vi "Actor Core.vi"(8 "error in":errorcluster, 11 "CS++GoBangClient in":refnum<class "CS++GoBangClient.lvclass">) -> (0 "error out":errorcluster, 3 "Actor out":refnum<class "Actor.lvclass">)   [LabVIEW 2013, in "GoBang.lvlib" / "CS++GoBangClient.lvclass"]
doc: "(<B>Filename</B>: Actor Framework.lvlib:Actor.lvclass:Actor Core.vi)\n\nReceives messages to the actor, reacts to them, and initiates any error handling that may shut the actor down.\n\nDescendant classes may override this VI to append parallel tasks for the actor to complete while it handles messages. Overrides use the Call Parent Method node."
uses:
  CS++GoBangClient.lvclass
  <vilib>/ActorFramework/Actor/Actor.lvclass
  typdefs/BoardField.ctl
  typdefs/GameState.ctl
  Core/Actors/CS++SVMonitor/CS++SVMonitor.lvclass
  CS++GoBangClient Messages/Write black player Msg/Write black player Msg.lvclass
  CS++GoBangClient Messages/Write white player Msg/Write white player Msg.lvclass
  CS++GoBangClient Messages/Write game board Msg/Write game board Msg.lvclass
  CS++GoBangClient Messages/Write game state Msg/Write game state Msg.lvclass
  Core/Actors/CS++BaseActor/CS++BaseActor.lvclass/CS++BaseActor.ctl
  <vilib>/ActorFramework/Actor/Actor.lvclass/Actor.ctl
  <vilib>/ActorFramework/Message Enqueuer/Message Enqueuer.lvclass/Message Enqueuer.ctl
  CS++GoBangClient.lvclass/CS++GoBangClient.ctl
  Core/Actors/CS++PVMonitor/CS++PVMonitor.lvclass/CS++PVMonitor.ctl
  Core/Actors/CS++PVMonitor Messages/Register PVs Msg/Register PVs Msg.lvclass/Register PVs Msg.ctl
  CS++GoBangClient Messages/Send Move Msg/Send Move Msg.lvclass/Send Move Msg.ctl
  CS++GoBangClient Messages/Join Game Msg/Join Game Msg.lvclass/Join Game Msg.ctl
  Core/Actors/CS++BaseActor/CS++BaseActor.lvclass
  <vilib>/ActorFramework/Message Enqueuer/Init from Existing Queue.vi
  <vilib>/ActorFramework/Message Enqueuer/Enqueue.vi
  <vilib>/ActorFramework/Message Priority Queue/Priority Enqueue.vi
  <vilib>/ActorFramework/Message Enqueuer/Message Enqueuer.lvclass
  Core/Actors/CS++PVMonitor Messages/Register PVs Msg/Register PVs Msg.lvclass
  CS++GoBangClient Messages/Send Move Msg/Send Move Msg.lvclass
  CS++GoBangClient Messages/Join Game Msg/Join Game Msg.lvclass
  <vilib>/ActorFramework/Stop Msg/Stop Msg.lvclass
  GoBang.lvlib
  Core/Actors/CS++PVMonitor/CS++PVMonitor.lvclass
  Core/Classes/CS++ProcessVariables/PVConnection/PVConnection.lvclass
panel:
  in  "OppColor":T1
  out "Opponnents name":string
  in  "Color":T1
  in  "Your name":string
  in  "stone":T1
  in  "stop":bool
  in  "State":T2
  out "GameBoard":T1[][](array[typedef])
  out "White won":bool
  out "Black won":bool
  out "Game over":bool
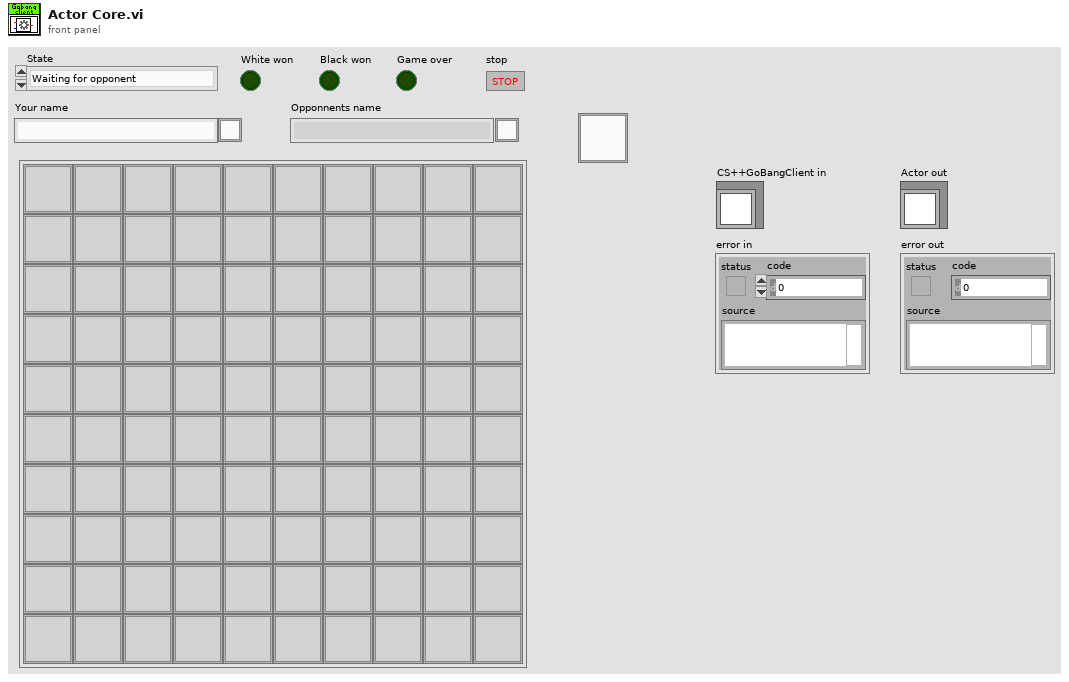
[diagram p1: front panel]
types:
  T1 = typedef "GoBang.lvlib/BoardField.ctl" = u8
  T2 = typedef "GoBang.lvlib/GameState.ctl" = enum16{"Waiting for opponent", "White to move", "Black to move", "Game over, white won", "Game over, black won"}
  T3 = enum32{"Invalid", "Standard", "Closed", "Hidden", "Minimized", "Maximized"}
  T4 = cluster{"BlackPlayer":string, "GoBang.lvlib:Write black player Msg.lvclass":refnum<class "Write black player Msg.lvclass">}
  T5 = cluster{"GameBoard":string, "GoBang.lvlib:Write game board Msg.lvclass":refnum<class "Write game board Msg.lvclass">}
  T6 = cluster{"GameState":string, "GoBang.lvlib:Write game state Msg.lvclass":refnum<class "Write game state Msg.lvclass">}
  T7 = cluster{"WhitePlayer":string, "GoBang.lvlib:Write white player Msg.lvclass":refnum<class "Write white player Msg.lvclass">}
  T8 = cluster{"GameState":string, "GoBang.lvlib:Write white player Msg.lvclass":refnum<class "CS++PVUpdate Msg.lvclass">}[]
  T9 = cluster{"Self Enqueuer":refnum<class "Message Enqueuer.lvclass">, cluster{"GameState":string, "GoBang.lvlib:Write white player Msg.lvclass":refnum<class "CS++PVUpdate Msg.lvclass">}[]}
  T10 = typedef "LVPositionTypeDef.ctl" = cluster{"Left":i32, "Top":i32}
  T11 = typedef "LVBoundsTypeDef.ctl" = cluster{"Width":u32, "Height":u32}
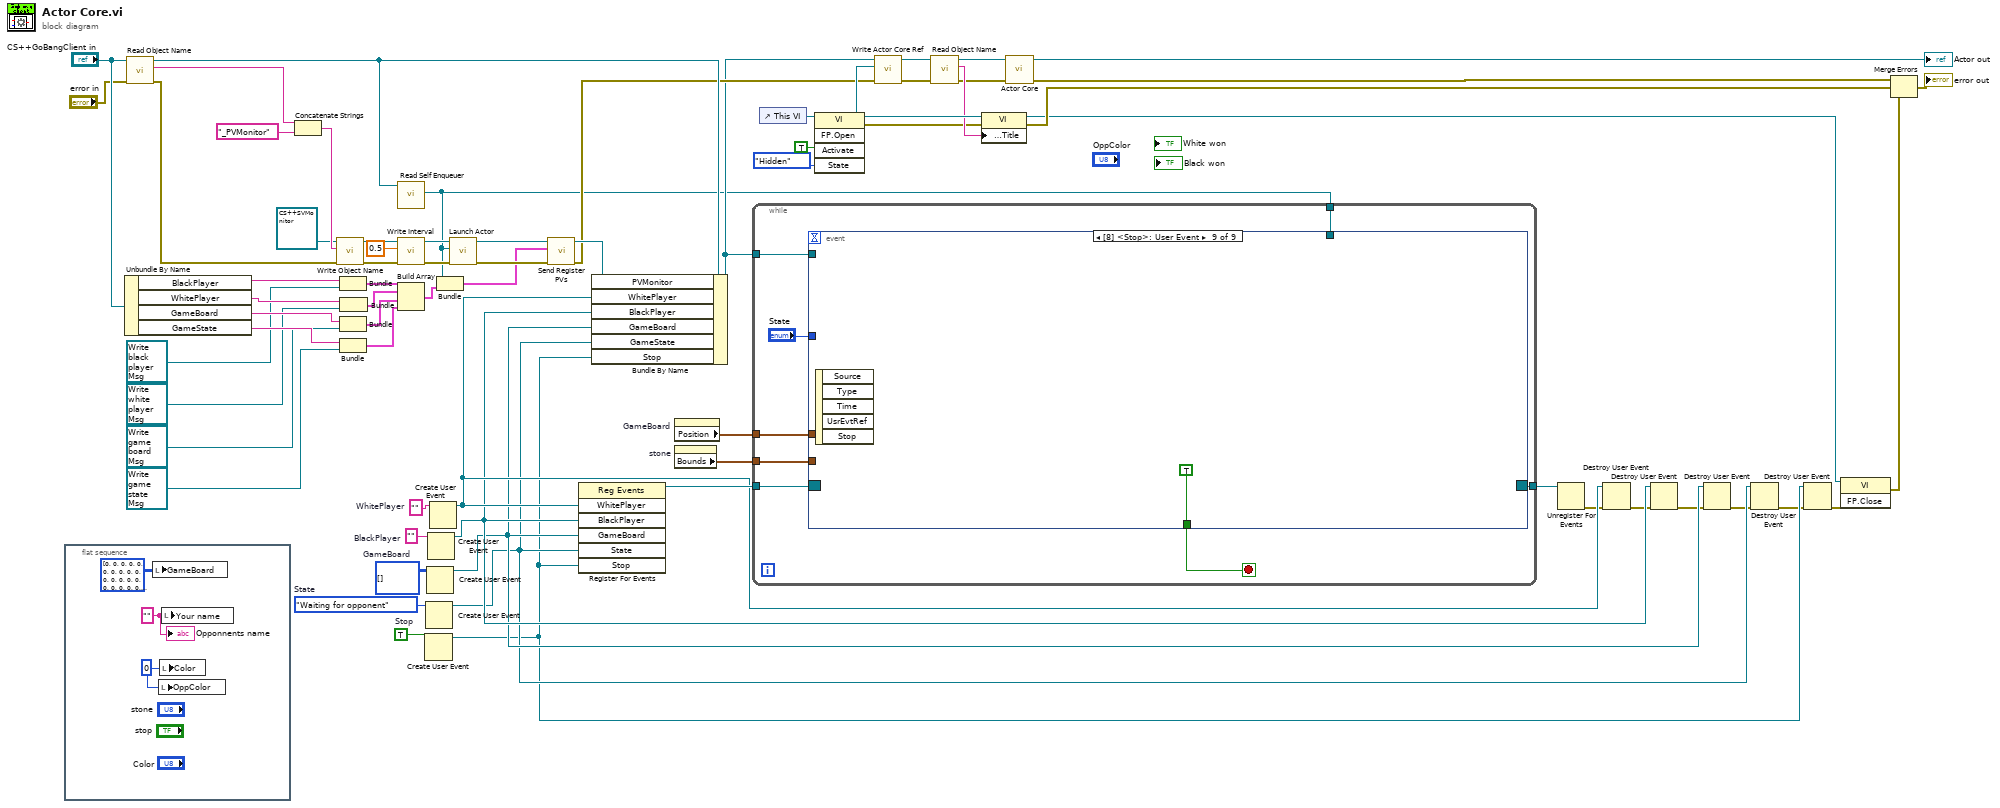
[diagram p0: block diagram]
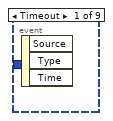
[diagram p2: hidden frame]
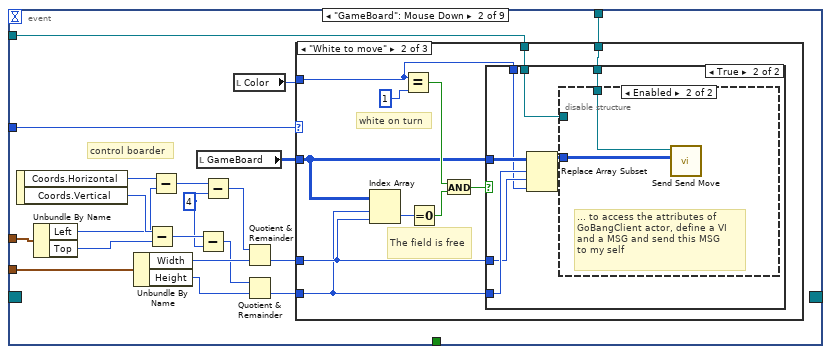
[diagram p3: hidden frame]
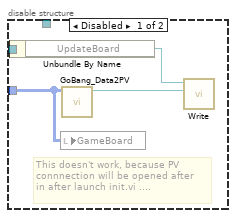
[diagram p6: hidden frame]
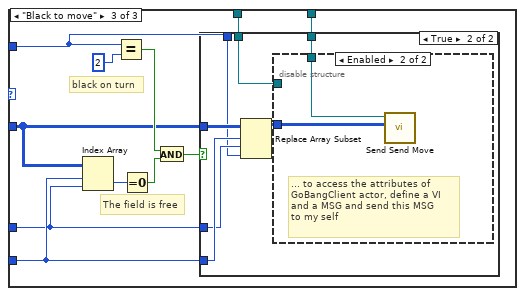
[diagram p7: hidden frame]
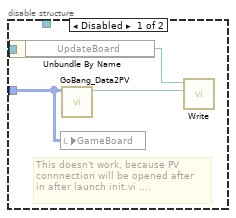
[diagram p9: hidden frame]
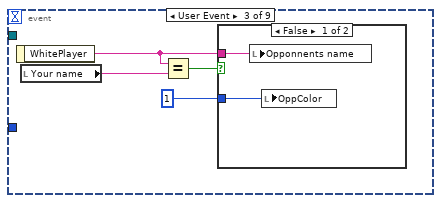
[diagram p10: hidden frame]
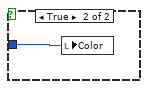
[diagram p11: hidden frame]
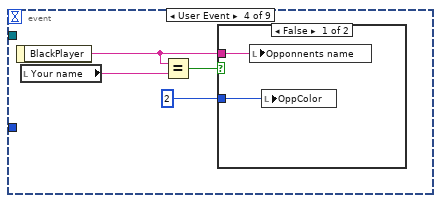
[diagram p12: hidden frame]
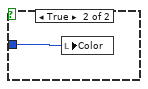
[diagram p13: hidden frame]
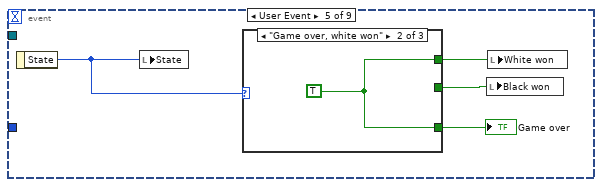
[diagram p14: hidden frame]
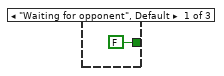
[diagram p15: hidden frame]
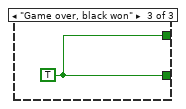
[diagram p16: hidden frame]
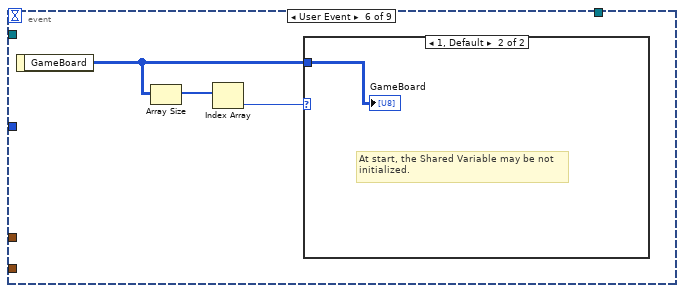
[diagram p17: hidden frame]
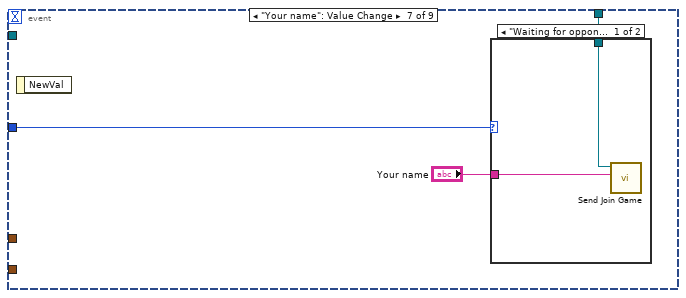
[diagram p19: hidden frame]
diagram:
  w32 = TRUE  # Stop
  w39 = T1[][] []  # GameBoard
  w40 = GameState."Waiting for opponent"  # State
  w41 = ""  # BlackPlayer
  w42 = ""  # WhitePlayer
  n1 = flat-sequence {
    frame #0 {
      w70 = T1 0 ("Color")
      w69 = "" ("Your name")
      n2 = local write "GameBoard"(T1[][] [[0, 0, 0, 0, 0, 0, 0, 0, 0, 0], [0, 0, 0, 0, 0, 0, 0, 0, 0, 0], [0, 0, 0, 0, 0, 0, 0, 0, 0, 0], [0, 0, 0, 0, 0, 0, 0, 0, 0, 0], [0, 0, 0, 0, 0, 0, 0, 0, 0, 0], [0, 0, 0, 0, 0, 0, 0, 0, 0, 0], [0, 0, 0, 0, 0, 0, 0, 0, 0, 0], [0, 0, 0, 0, 0, 0, 0, 0, 0, 0], [0, 0, 0, 0, 0, 0, 0, 0, 0, 0], [0, 0, 0, 0, 0, 0, 0, 0, 0, 0]] ("GameBoard")) -> ()
      n3 = local write "OppColor"(w70) -> ()
      n4 = local write "Color"(w70) -> ()
      n5 = local write "Your name"(w69) -> ()
      "Opponnents name" <- w69
    }
  }
  n6 = Unbundle By Name("CS++GoBangClient in") -> ("BlackPlayer"=w64:string, "WhitePlayer"=w48:string, "GameBoard"=w47:string, "GameState"=w46:string)
  n7 = call "Read Object Name.vi"("error in (no error)"="error in", "CS++BaseActor in"="CS++GoBangClient in") -> ("error out"=w19:errorcluster, "Object Name"=w50:string, "CS++BaseActor out"=w33:refnum<class "CS++GoBangClient.lvclass">)  [unwired: 7 in]
  n8 = Concatenate Strings(w50, "_PVMonitor" ("Object Name")) -> (w58:string)
  n9 = call "Write Object Name.vi"("error in (no error)"=w19, "Object Name"=w58, "CS++BaseActor in"=refnum<class "CS++SVMonitor.lvclass"> refnum ("CS++SVMonitor.lvlib:CS++SVMonitor.lvclass")) -> ("error out"=w55:errorcluster, "CS++BaseActor out"=w57:refnum<class "CS++SVMonitor.lvclass">)  [unwired: 7 in]
  n10 = Bundle("BlackPlayer"=w64, "GoBang.lvlib:Write black player Msg.lvclass"=refnum<class "Write black player Msg.lvclass"> refnum) -> (w63:T4)  [unwired: 1 in]
  n11 = Bundle("GameBoard"=w47, "GoBang.lvlib:Write game board Msg.lvclass"=refnum<class "Write game board Msg.lvclass"> refnum) -> (w44:T5)  [unwired: 1 in]
  n12 = Bundle("GameState"=w46, "GoBang.lvlib:Write game state Msg.lvclass"=refnum<class "Write game state Msg.lvclass"> refnum) -> (w43:T6)  [unwired: 1 in]
  n13 = Bundle("WhitePlayer"=w48, "GoBang.lvlib:Write white player Msg.lvclass"=refnum<class "Write white player Msg.lvclass"> refnum) -> (w45:T7)  [unwired: 1 in]
  n14 = call <vilib>:"Read Self Enqueuer.vi"("Actor"=w33) -> ("Self Enqueuer"=w5:refnum<class "Message Enqueuer.lvclass">)  [unwired: 10 in]
  n15 = call "Write Interval.vi"("error in (no error)"=w55, "Interval"=dbl[unit] 0.5, "CS++PVMonitor in"=w57) -> ("error out"=w51:errorcluster, "CS++PVMonitor out"=w59:refnum<class "CS++SVMonitor.lvclass">)  [unwired: 7 in]
  n16 = Build Array(w63, w45, w44, w43) -> (w62:T8)
  n17 = Create User Event(user event datatype=w32) -> (user event=w12:refnum<user-event>)  [unwired: 1 in, 1 out]
  n18 = Create User Event(user event datatype=w40) -> (user event=w13:refnum<user-event>)  [unwired: 1 in, 1 out]
  n19 = Create User Event(user event datatype=w39) -> (user event=w14:refnum<user-event>)  [unwired: 1 in, 1 out]
  n20 = Create User Event(user event datatype=w41) -> (user event=w15:refnum<user-event>)  [unwired: 1 in, 1 out]
  n21 = Create User Event(user event datatype=w42) -> (user event=w16:refnum<user-event>)  [unwired: 1 in, 1 out]
  n22 = Bundle("Self Enqueuer"=w5, w62) -> (w53:T9)  [unwired: 1 in]
  n23 = call <vilib>:"Launch Actor.vi"("error in (no error)"=w51, "Actor-to-Caller Enqueuer"=w5, "Actor"=w59) -> ("error out"=w54:errorcluster, "Caller-To-Actor Enqueuer"=w52:refnum<class "Message Enqueuer.lvclass">)  [unwired: 7 in]
  n24 = call "Send Register PVs.vi"("error in (no error)"=w54, "Register Info"=w53, "Message Enqueuer"=w52) -> ("error out"=w18:errorcluster)  [unwired: 7 in, 1 out]
  n25 = register-events(w16, w15, w14, w13, w12) -> (reference out=w38:refnum<event-registration>)  [unwired: 2 in, 1 out]
  n26 = Bundle By Name(cluster=w33, "PVMonitor"=w52, "WhitePlayer"=w16, "BlackPlayer"=w15, "GameBoard"=w14, "GameState"=w13, "Stop"=w12) -> (w6:refnum<class "CS++GoBangClient.lvclass">)
  n27 = property on="GameBoard" class="Arr (strict)"() -> ("Position"=w65:T10)  [unwired: 2 in, 2 out]
  n28 = property on="stone" class="Ring (strict)"() -> ("Bounds"=w66:T11)  [unwired: 2 in, 2 out]
  n29 = while {
    tunnel: w66 -> [w78]
    tunnel: w65 -> [w77]
    tunnel: w38 -> [w76]
    tunnel: w6 -> [w75]
    tunnel: [w73] -> w17
    tunnel: w5 -> [w72]
    stop <- w79 stop-if-true
    n30 = event shown="[8] <Stop>: User Event" {
      selector: w76 -> [_ _ _ _ _ _ _ _ _]
      dyn-events: [_ _ _ _ _ _ _ _ _] -> w73
      timeout: _ -> [_ _ _ _ _ _ _ _ _]
      tunnel: [_ _ _ _ _ _ _ TRUE TRUE] -> w79
      tunnel: w78 -> [_ w99 _ _ _ _ _ _ _]
      tunnel: w77 -> [_ w94 _ _ _ _ _ _ _]
      tunnel: w75 -> [_ w81 _ _ _ _ _ w180 _]
      tunnel: "State" -> [_ w84 _ _ _ _ w175 _ _]
      tunnel: w72 -> [_ w80 _ _ _ _ w173 _ _]
      event Timeout {
        n31 = event-data() -> ()  [unwired: 1 in, 3 out]
      }
      event "GameBoard": Mouse Down {
        w87 = 4 ("y 2")
        # "control boarder"
        n32 = event-data() -> ("Coords.Horizontal"=w98:i32, "Coords.Vertical"=w96:i32)  [unwired: 1 in]
        n33 = Unbundle By Name(w94) -> ("Left"=w93:i32, "Top"=w92:i32)
        n34 = Unbundle By Name(w99) -> ("Width"=w97:u32, "Height"=w95:u32)
        n35 = Subtract(x=w96, y=w92) -> (x-y=w90:i32)
        n36 = Subtract(x=w98, y=w93) -> (x-y=w91:i32)
        n37 = local read "GameBoard"() -> (w83:T1[][])
        n38 = Subtract(x=w90, y=w87) -> (x-y=w88:i32)
        n39 = Subtract(x=w91, y=w87) -> (x-y=w89:i32)
        n40 = local read "Color"() -> (w82:T1)
        n41 = Quotient & Remainder(x=w89, y=w97) -> (floor(x/y)=w86:u32)  [unwired: 1 out]
        n42 = Quotient & Remainder(x=w88, y=w95) -> (floor(x/y)=w85:u32)  [unwired: 1 out]
        n43 = case shown="\"White to move\"" w84 {
          tunnel: w86 -> [_ w102 w133]
          tunnel: w85 -> [_ w101 w134]
          tunnel: w83 -> [_ w104 w128]
          tunnel: w82 -> [_ w100 w126]
          tunnel: w81 -> [_ w105 w125]
          tunnel: w80 -> [_ w106 w124]
          frame "Waiting for opponent", Default {
          }
          frame "White to move" {
            # "white on turn"
            # "The field is free"
            n44 = Index Array(array=w104, index (row)=w101, index (col)=w102) -> (element=w110:T1)
            n45 = Equal?(x=w100, y=T1 1) -> (x = y?=w108:bool)
            n46 = Equal To 0?(x=w110) -> (x = 0?=w109:bool)
            n47 = And(x=w108, y=w109) -> (x .and. y?=w103:bool)
            n48 = case shown="True" w103 {
              tunnel: w101 -> [_ w117]
              tunnel: w102 -> [_ w116]
              tunnel: w104 -> [_ w115]
              tunnel: w100 -> [_ w114]
              tunnel: w105 -> [_ w112]
              tunnel: w106 -> [_ w111]
              frame False {
              }
              frame True {
                n49 = Replace Array Subset(array=w115, new element=w114, index (row)=w117, index (col)=w116) -> (w113:T1[][])
                n50 = disable-structure shown="Enabled" {
                  disable-tunnel: w113 -> [w120 w122]
                  disable-tunnel: w112 -> [w118 _]
                  disable-tunnel: w111 -> [_ w123]
                  frame Disabled {
                    # "This doesn't work, because PV\nconnnection will be opened after\nin after launch init.vi ...."
                    n51 = Unbundle By Name(w118) -> ("UpdateBoard"=w119:refnum<class "PVConnection.lvclass">)
                    n52 = local write "GameBoard"(w120) -> ()
                    n53 = call "GoBang_Data2PV.vi"("Data in"=w120) -> ("PV out"=w121:refnum<class "PV.lvclass">)  [unwired: 10 in]
                    n54 = call-dynamic "Write.vi"("PV"=w121, "PVConnection in"=w119) -> ()  [unwired: 8 in, 2 out]
                  }
                  frame Enabled {
                    # "... to access the attributes of \nGoBangClient actor, define a VI \nand a MSG and send this MSG \nto my self"
                    n55 = call "Send Send Move.vi"("GameBoard"=w122, "Message Enqueuer"=w123) -> ()  [unwired: 8 in, 2 out]
                  }
                }
              }
            }
          }
          frame "Black to move" {
            # "black on turn"
            # "The field is free"
            n56 = Index Array(array=w128, index (row)=w134, index (col)=w133) -> (element=w132:T1)
            n57 = Equal?(x=w126, y=T1 2) -> (x = y?=w129:bool)
            n58 = Equal To 0?(x=w132) -> (x = 0?=w130:bool)
            n59 = And(x=w129, y=w130) -> (x .and. y?=w131:bool)
            n60 = case shown="True" w131 {
              tunnel: w134 -> [_ w141]
              tunnel: w133 -> [_ w140]
              tunnel: w128 -> [_ w139]
              tunnel: w126 -> [_ w138]
              tunnel: w125 -> [_ w136]
              tunnel: w124 -> [_ w135]
              frame False {
              }
              frame True {
                n61 = Replace Array Subset(array=w139, new element=w138, index (row)=w141, index (col)=w140) -> (w137:T1[][])
                n62 = disable-structure shown="Enabled" {
                  disable-tunnel: w137 -> [w144 w146]
                  disable-tunnel: w136 -> [w142 _]
                  disable-tunnel: w135 -> [_ w147]
                  frame Disabled {
                    # "This doesn't work, because PV\nconnnection will be opened after\nin after launch init.vi ...."
                    n63 = Unbundle By Name(w142) -> ("UpdateBoard"=w143:refnum<class "PVConnection.lvclass">)
                    n64 = local write "GameBoard"(w144) -> ()
                    n65 = call "GoBang_Data2PV.vi"("Data in"=w144) -> ("PV out"=w145:refnum<class "PV.lvclass">)  [unwired: 10 in]
                    n66 = call-dynamic "Write.vi"("PV"=w145, "PVConnection in"=w143) -> ()  [unwired: 8 in, 2 out]
                  }
                  frame Enabled {
                    # "... to access the attributes of \nGoBangClient actor, define a VI \nand a MSG and send this MSG \nto my self"
                    n67 = call "Send Send Move.vi"("GameBoard"=w146, "Message Enqueuer"=w147) -> ()  [unwired: 8 in, 2 out]
                  }
                }
              }
            }
          }
        }
      }
      event User Event {
        n68 = event-data() -> ("WhitePlayer"=w149:string)  [unwired: 1 in]
        n69 = local read "Your name"() -> (w151:string)
        n70 = Equal?(x=w149, y=w151) -> (x = y?=w150:bool)
        n71 = case shown="False" w150 {
          tunnel: w149 -> [w153 _]
          tunnel: T1 1 ("Color") -> [w152 w154]
          frame False {
            n72 = local write "Opponnents name"(w153) -> ()
            n73 = local write "OppColor"(w152) -> ()
          }
          frame True {
            n74 = local write "Color"(w154) -> ()
          }
        }
      }
      event User Event {
        n75 = event-data() -> ("BlackPlayer"=w156:string)  [unwired: 1 in]
        n76 = local read "Your name"() -> (w158:string)
        n77 = Equal?(x=w156, y=w158) -> (x = y?=w157:bool)
        n78 = case shown="False" w157 {
          tunnel: w156 -> [w160 _]
          tunnel: T1 2 ("Color") -> [w159 w161]
          frame False {
            n79 = local write "Opponnents name"(w160) -> ()
            n80 = local write "OppColor"(w159) -> ()
          }
          frame True {
            n81 = local write "Color"(w161) -> ()
          }
        }
      }
      event User Event {
        n82 = event-data() -> ("State"=w165:T2)  [unwired: 1 in]
        n83 = local write "State"(w165) -> ()
        n84 = case shown="\"Waiting for opponent\", Default" w165 {
          tunnel: [FALSE ("White won") w167 w168] -> w164
          tunnel: [_ _ w168] -> w163
          tunnel: [_ w167 _] -> w162
          frame "Waiting for opponent", Default {
          }
          frame "Game over, white won" {
            w167 = TRUE ("White won")
          }
          frame "Game over, black won" {
            w168 = TRUE ("White won")
          }
        }
        "Game over" <- w164
        n85 = local write "Black won"(w163) -> ()
        n86 = local write "White won"(w162) -> ()
      }
      event User Event {
        n87 = event-data() -> ("GameBoard"=w169:T1[][])  [unwired: 1 in]
        n88 = Array Size(array=w169) -> (size(s)=w171:i32[])
        n89 = Index Array(array=w171) -> (element=w170:i32)  [unwired: 1 in]
        n90 = case shown="1, Default" w170 {
          tunnel: w169 -> [_ w172]
          frame 0 {
          }
          frame 1, Default {
            # "At start, the Shared Variable may be not\ninitialized."
            "GameBoard" <- w172
          }
        }
      }
      event "Your name": Value Change {
        n91 = event-data() -> ()  [unwired: 1 in, 1 out]
        n92 = case shown="\"Waiting for opponent\"" w175 {
          tunnel: "Your name" -> [w176 _]
          tunnel: w173 -> [w177 _]
          frame "Waiting for opponent" {
            n93 = call "Send Join Game.vi"("Your name"=w176, "Message Enqueuer"=w177) -> ()  [unwired: 8 in, 2 out]
          }
          frame "White to move", Default {
          }
        }
      }
      event "stop": Mouse Down {
        n94 = event-data() -> ()  [unwired: 1 in, 1 out]
        n95 = call <vilib>:"Read Self Enqueuer.vi"("Actor"=w180) -> ("Self Enqueuer"=w178:refnum<class "Message Enqueuer.lvclass">)  [unwired: 10 in]
        n96 = call <vilib>:"Send Normal Stop.vi"("Message Enqueuer"=w178) -> ("error out"=w179:errorcluster)  [unwired: 10 in]
        n97 = call <vilib>:"Simple Error Handler.vi"("error in (no error)"=w179) -> ()  [unwired: 4 in, 5 out]
      }
      event User Event {
        n98 = event-data() -> ()  [unwired: 1 in, 5 out]
      }
    }
  }
  n99 = control-ref of="This VI"() -> (w29:refnum<vi>)
  n100 = invoke class="VI" method="FP.Open"(reference=w29, "Activate"=TRUE ("Activate?"), "State"=T3."Hidden") -> (reference out=w26:refnum<vi>, error out=w21:errorcluster)  [unwired: 2 in, 3 out]
  n101 = call "Write Actor Core Ref.vi"("error in (no error)"=w18, "Actor Core Ref"=w26, "CS++BaseActor in"=w6) -> ("error out"=w27:errorcluster, "CS++BaseActor out"=w28:refnum<class "CS++GoBangClient.lvclass">)  [unwired: 7 in]
  n102 = call "Read Object Name.vi"("error in (no error)"=w27, "CS++BaseActor in"=w28) -> ("error out"=w23:errorcluster, "Object Name"=w25:string, "CS++BaseActor out"=w24:refnum<class "CS++GoBangClient.lvclass">)  [unwired: 7 in]
  n103 = property class="VI"(reference=w26, error in=w21, "Front Panel.Title"=w25) -> (reference out=w3:refnum<vi>, error out=w20:errorcluster)
  n104 = call-parent "Actor Core.vi"("error in"=w23, "CS++BaseActor in"=w24) -> ("error out"=w68:errorcluster, "Actor out"=→"Actor out":refnum<class "Actor.lvclass">)  [unwired: 8 in]
  n105 = Unregister For Events(event registration refnum=w17) -> (error out=w11:errorcluster)  [unwired: 1 in]
  n106 = Destroy User Event(user event=w16, error in=w11) -> (error out=w10:errorcluster)
  n107 = Destroy User Event(user event=w15, error in=w10) -> (error out=w9:errorcluster)
  n108 = Destroy User Event(user event=w14, error in=w9) -> (error out=w8:errorcluster)
  n109 = Destroy User Event(user event=w13, error in=w8) -> (error out=w7:errorcluster)
  n110 = Destroy User Event(user event=w12, error in=w7) -> (error out=w4:errorcluster)
  n111 = invoke class="VI" method="FP.Close"(reference=w3, error in=w4) -> (error out=w1:errorcluster)  [unwired: 1 in, 2 out]
  n112 = Merge Errors(w68, w20, w1) -> (→"error out":errorcluster)
